vi "Get_dR_dX_dY-1.vi"(3 "Y2":dbl, 4 "X2":dbl, 5 "Y1":dbl, 6 "X1":dbl) -> (0 "dR":dbl, 1 "dY":dbl, 2 "dX":dbl)   [LabVIEW 2013]
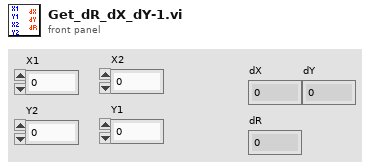
[diagram p1: front panel]
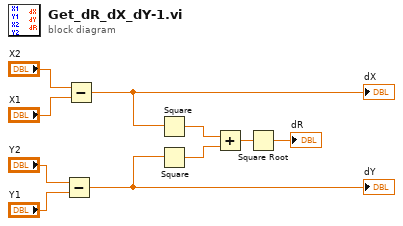
[diagram p0: block diagram]
diagram:
  n1 = Subtract(x="Y2", y="Y1") -> (x-y=w5:dbl)
  "dY" <- w5
  n2 = Subtract(x="X2", y="X1") -> (x-y=w6:dbl)
  "dX" <- w6
  n3 = Square(x=w6) -> (x^2=w4:dbl)
  n4 = Square(x=w5) -> (x^2=w3:dbl)
  n5 = Add(x=w4, y=w3) -> (x+y=w2:dbl)
  n6 = Square Root(x=w2) -> (sqrt(x)=→"dR":dbl)
